vi "Initialize.vi"(6 "optional":variant, 8 "error in":errorcluster, 11 "Categories in":refnum<class "Categories.lvclass">) -> (0 "error out":errorcluster, 3 "Node*":refnum<data-value>)   [LabVIEW 2013, in "Categories.lvclass"]
doc: "Initializes a node. Makes a data value reference of the node, sets the selfNode, and output the data value reference."
uses:
  Categories.lvclass
  xCE/xceNode/xceNode.lvclass
  xCE/xceDataNode/xceDataNode.lvclass
  Category/Category.lvclass
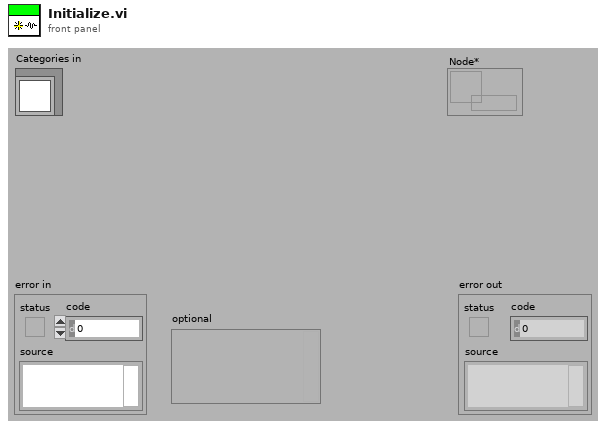
[diagram p1: front panel]
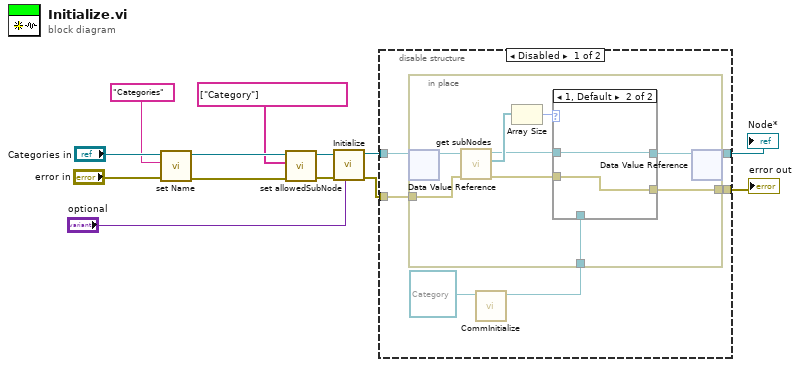
[diagram p0: block diagram]
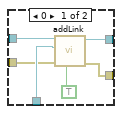
[diagram p2: hidden frame]
diagram:
  n1 = call "set Name.vi"("error in (no error)"="error in", "Name"="Categories", "xceDataNode in"="Categories in") -> ("error out"=w9:errorcluster, "xceDataNode out"=w8:refnum<class "Categories.lvclass">)  [unwired: 7 in]
  n2 = call "set allowedSubNode.vi"("error in (no error)"=w9, "Allowed subNode[]"=string[] ["Category"], "xceDataNode in"=w8) -> ("error out"=w5:errorcluster, "xceDataNode out"=w6:refnum<class "Categories.lvclass">)  [unwired: 7 in]
  n3 = call-parent "Initialize.vi"("optional"="optional", "error in"=w5, "xceDataNode in"=w6) -> ("error out"=w3:errorcluster, "Node*"=w4:refnum<data-value>)  [unwired: 7 in]
  n4 = disable-structure shown="Disabled" {
    disable-tunnel: w4 -> [w19 w38]
    disable-tunnel: w3 -> [w18 w37]
    disable-tunnel: [w17 w37] -> w2
    disable-tunnel: [w16 w38] -> w1
    frame Disabled {
      n5 = call "CommInitialize.vi"("Category in"=refnum<class "Category.lvclass"> refnum) -> ("Node*"=w14:refnum<data-value>)  [unwired: 9 in, 1 out]
      n6 = in-place {
        in-place-border: w14 -> [w27]
        in-place-border: w18 -> [w22]
        in-place-border: [w26] -> w17
        n7 = in-place-dvr #1(w19) -> (w25:refnum<class "xceNode.lvclass">)  [unwired: 1 out]
        n8 = call "get subNodes.vi"("error in (no error)"=w22, "xceNode in"=w25) -> ("error out"=w21:errorcluster, "subNodes[]*"=w24:refnum<data-value>[], "xceNode out"=w23:refnum<class "xceNode.lvclass">)  [unwired: 7 in]
        n9 = Array Size(array=w24) -> (size(s)=w20:i32)
        n10 = case shown="1, Default" w20 {
          tunnel: [w33 w36] -> w28
          tunnel: w27 -> [w32 _]
          tunnel: [w31 w35] -> w26
          tunnel: w23 -> [w30 w36]
          tunnel: w21 -> [w29 w35]
          frame 0 {
            n11 = call "addLink.vi"("Append to End"=TRUE, "error in (no error)"=w29, "subNode in"=w32, "superNode in"=w30) -> ("error out"=w31:errorcluster, "superNode out"=w33:refnum<class "xceNode.lvclass">)  [unwired: 5 in, 1 out]
          }
          frame 1, Default {
          }
        }
        n12 = in-place-dvr #1(w28) -> (w16:refnum<data-value>)  [unwired: 1 out]
      }
    }
    frame Enabled {
    }
  }
  "error out" <- w2
  "Node*" <- w1
